vi "GetText.vi"(8 "error in (no error)":errorcluster, 11 "reference in":refnum<class "Text.lvclass">) -> (0 "error out":errorcluster, 2 "Text":string, 3 "reference out":refnum<class "Text.lvclass">)   [LabVIEW 2010, in "Labricks.lvlib" / "Text.lvclass"]
uses:
  Text.lvclass
  RenderBase/SceneObject_class/SceneObject.lvclass
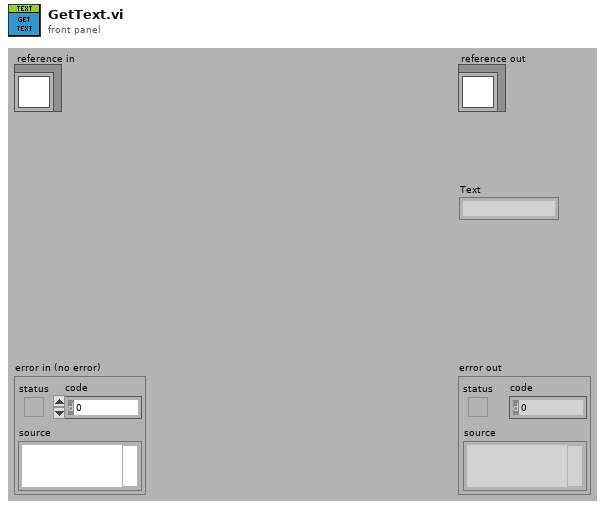
[diagram p1: front panel]
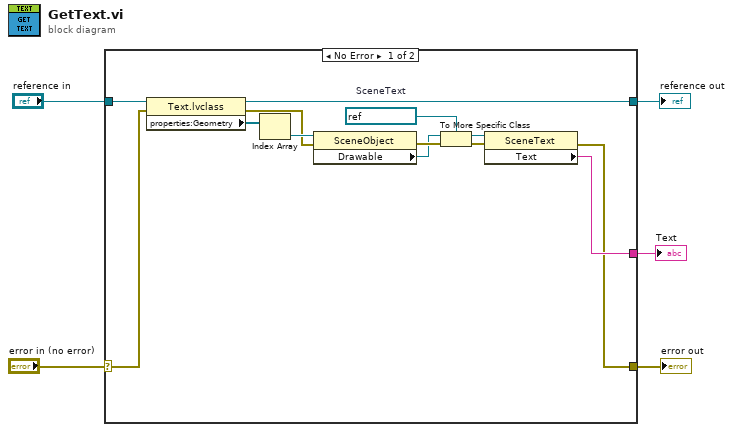
[diagram p0: block diagram]
diagram:
  n1 = case shown="No Error" "error in (no error)" {
    selector: "error in (no error)" -> [w11 w20]
    tunnel: [w9 w20] -> w4
    tunnel: [w17 w19] -> w2
    tunnel: "reference in" -> [w18 w19]
    tunnel: [w10 _] -> w1
    frame No Error {
      w14 = refnum<vi> refnum  # SceneText
      n2 = property class="Text.lvclass"(reference=w18, error in=w11) -> (reference out=w17:refnum<class "Text.lvclass">, error out=w8:errorcluster, "properties:Geometry"=w16:refnum<vi>[])
      n3 = Index Array(array=w16) -> (element=w15:refnum<vi>)  [unwired: 1 in]
      n4 = property class="SceneObject"(reference=w15, error in=w8) -> (error out=w7:errorcluster, "Drawable"=w6:refnum<vi>)  [unwired: 1 out]
      n5 = To More Specific Class(target class=w14, reference=w6, error in=w7) -> (specific class reference=w13:refnum<vi>, error out=w12:errorcluster)
      n6 = property class="SceneText"(reference=w13, error in=w12) -> (error out=w9:errorcluster, "Text"=w10:string)  [unwired: 1 out]
    }
    frame Error {
    }
  }
  "error out" <- w4
  "reference out" <- w2
  "Text" <- w1
